vi "Element Type.vi"(11 "2WayValve in":refnum<class "2WayValveV.lvclass">) -> (2 "Control Type":string)   [LabVIEW 2020, in "VolatusGUIElements.lvlib" / "2WayValveV.lvclass"]
uses:
  2WayValveV.lvclass
  2WayValveV.lvclass/2WayValveV.ctl
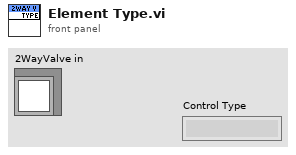
[diagram p1: front panel]
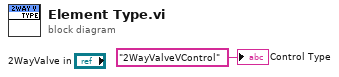
[diagram p0: block diagram]
diagram:
  "Control Type" <- "2WayValveVControl" ("Control Type")
